vi "Start Measurement.vi"(8 "error in (no error)":errorcluster, 11 "Keithley electrometer in":refnum<class "Keithley electrometer.lvclass">) -> (0 "error out":errorcluster, 3 "Keithley electrometer out":refnum<class "Keithley electrometer.lvclass">)   [LabVIEW 2015, in "Keithley electrometer.lvclass"]
uses:
  Keithley electrometer.lvclass
  Meter/Keithley Meter Parameters.ctl
  Meter/KeithleyMeter Function.ctl
  Instrument/Read VISA Resource.vi
  OO Devices/Device/Read Controls Snapshot.vi
  Instrument/Write VISA Resource.vi
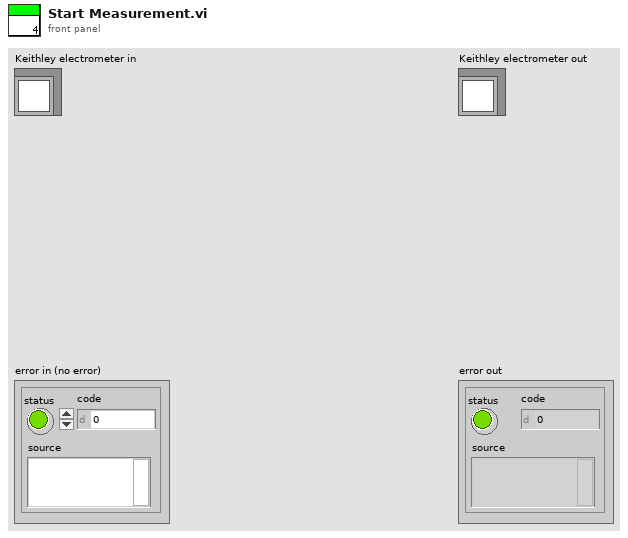
[diagram p1: front panel]
types:
  T1 = typedef "Keithley Meter Parameters.ctl" = cluster{"Range (-1: auto)":dbl, "Integration Time (NPLCs)":dbl, "Function":T2, "W Offset comp":bool, "4-wire W":bool, "Scale":dbl, "Offset":dbl}
  T2 = typedef "KeithleyMeter Function.ctl" = enum16{"VOLTAGE", "CURRENT", "RESISTANCE"}
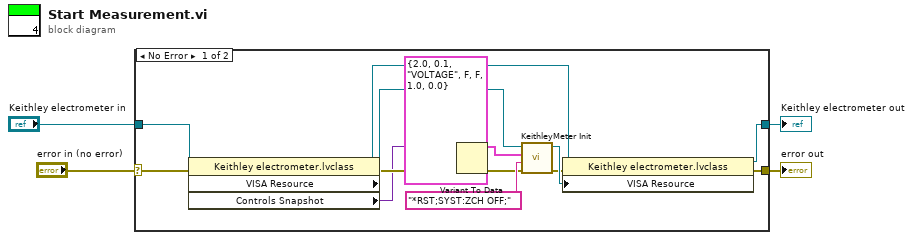
[diagram p0: block diagram]
diagram:
  n1 = case shown="No Error" "error in (no error)" {
    selector: "error in (no error)" -> [w12 w20]
    tunnel: [w5 w20] -> w3
    tunnel: [w16 w19] -> w1
    tunnel: "Keithley electrometer in" -> [w18 w19]
    frame No Error {
      n2 = property class="Keithley electrometer.lvclass"(reference=w18, error in=w12) -> (reference out=w17:refnum<class "Keithley electrometer.lvclass">, error out=w11:errorcluster, "VISA Resource"=w13:refnum<visa-resource-name>, "Controls Snapshot"=w10:variant)
      n3 = Variant To Data(error in=w11, type=T1 {"Range (-1: auto)"=2.0, "Integration Time (NPLCs)"=0.1, "Function"=enum."VOLTAGE", "W Offset comp"=FALSE, "4-wire W"=FALSE, "Scale"=1.0, "Offset"=0.0} ("Parameters"), Variant=w10) -> (data=w8:T1, error out=w7:errorcluster)
      n4 = call "KeithleyMeter Init.vi"("Error In"=w7, "Prefix command"="*RST;SYST:ZCH OFF;" ("write buffer"), "Parameters"=w8, "VISA resource name"=w13) -> ("Error Out"=w6:errorcluster, "VISA resource name out"=w15:refnum<visa-resource-name>)  [unwired: 6 in]
      n5 = property class="Keithley electrometer.lvclass"(reference=w17, error in=w6, "VISA Resource"=w15) -> (reference out=w16:refnum<class "Keithley electrometer.lvclass">, error out=w5:errorcluster)
    }
    frame Error {
    }
  }
  "error out" <- w3
  "Keithley electrometer out" <- w1
